vi "CallVIs.vi"(2 "error in (no error)":errorcluster, 3 "Queues":T1[](array[typedef])) -> (0 "error out":errorcluster)   [LabVIEW 2018]
uses:
  <vilib>/NI/AMC/Message Queue.ctl
  <vilib>/NI/AMC/Message.ctl
  <vilib>/NI/Tools/Keyed Array/KeyedArray.ctl
  QueueNames.ctl
  <vilib>/NI/Tools/Keyed Array/Tools_KeyedArray.lvlib
  <vilib>/NI/AMC/AMC.lvlib
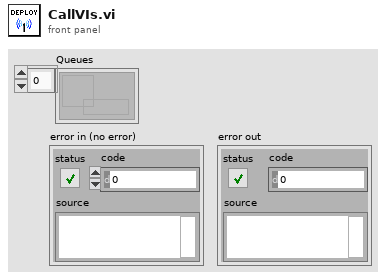
[diagram p1: front panel]
types:
  T1 = typedef "AMC.lvlib/Message Queue.ctl" = refnum<queue>
  T2 = typedef "QueueNames.ctl" = enum32{"Handler", "RT Loop", "Slow AO"}
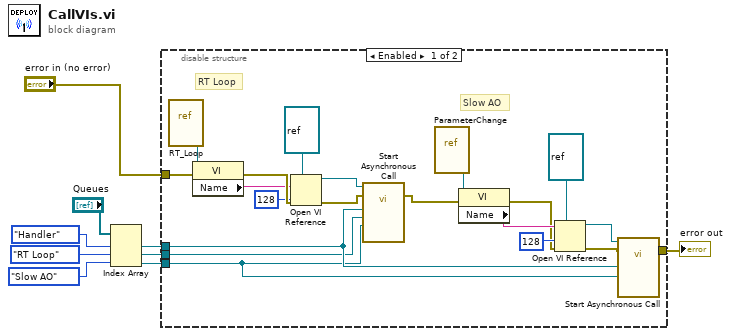
[diagram p0: block diagram]
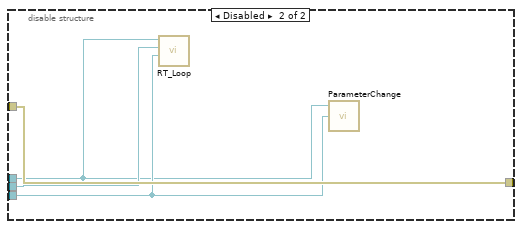
[diagram p2: hidden frame]
diagram:
  n1 = Index Array(array="Queues", index #1=QueueNames."Handler" ("Queue Name Refs"), index #2=QueueNames."RT Loop" ("Queue Name Refs"), index #3=QueueNames."Slow AO" ("Queue Name Refs")) -> (element #1=w3:T1, element #2=w2:T1, element #3=w1:T1)
  n2 = disable-structure shown="Enabled" {
    disable-tunnel: "error in (no error)" -> [w19 w33]
    disable-tunnel: [w15 w33] -> w4
    disable-tunnel: w3 -> [w12 w30]
    disable-tunnel: w2 -> [w11 w31]
    disable-tunnel: w1 -> [w10 w32]
    frame Enabled {
      # "Slow AO"
      # "RT Loop"
      n3 = vi-ref "RT_Loop.vi"() -> (w25:refnum<vi>)
      n4 = property class="VI"(reference=w25, error in=w19) -> (error out=w29:errorcluster, "Name"=w26:string)  [unwired: 1 out]
      n5 = Open VI Reference(type specifier VI Refnum (for type only)=refnum<vi> refnum, vi path=w26, options=128, error in (no error)=w29) -> (vi reference=w17:refnum<vi>, error out=w18:errorcluster)  [unwired: 2 in]
      n6 = call-by-ref "Start Asynchronous Call"(reference=w17, error in=w18, "Param Qname"=w10, "RT Loop Qname"=w11, "Handler Qname"=w12) -> (error out=w16:errorcluster)  [unwired: 1 in, 1 out]
      n7 = vi-ref "ParameterChange.vi"() -> (w24:refnum<vi>)
      n8 = property class="VI"(reference=w24, error in=w16) -> (error out=w20:errorcluster, "Name"=w23:string)  [unwired: 1 out]
      n9 = Open VI Reference(type specifier VI Refnum (for type only)=refnum<vi> refnum, vi path=w23, options=128, error in (no error)=w20) -> (vi reference=w13:refnum<vi>, error out=w14:errorcluster)  [unwired: 2 in]
      n10 = call-by-ref "Start Asynchronous Call"(reference=w13, error in=w14, "Slow AO Qname"=w10, "Handler Qname"=w12) -> (error out=w15:errorcluster)  [unwired: 3 in, 1 out]
    }
    frame Disabled {
      n11 = call "RT_Loop.vi"("Param Qname"=w32, "RT Loop Qname"=w31, "Handler Qname"=w30) -> ()  [unwired: 1 in]
      n12 = call "ParameterChange.vi"("Slow AO Qname"=w32, "Handler Qname"=w30) -> ()  [unwired: 3 in]
    }
  }
  "error out" <- w4
